vi "Generate And Open Html.vi"(8 "error in":errorcluster, 10 "Generated File Path":path, 11 "Open Generated Document":bool=TRUE) -> (0 "error out":errorcluster)   [LabVIEW 2019, in "Panther Dashboard.lvlib"]
uses:
  Panther Dashboard.lvlib
  <vilib>/Wovalab/AsciiDoc for LabVIEW/Output Format--enum.ctl
  <vilib>/Wovalab/AsciiDoc for LabVIEW/Wovalab_lib_AsciiDoctor.lvlib
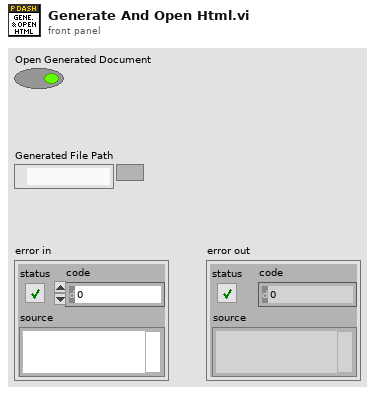
[diagram p1: front panel]
types:
  T1 = typedef "Wovalab_lib_AsciiDoctor.lvlib/Output Format--enum.ctl" = enum16{"HTML5", "PDF"}
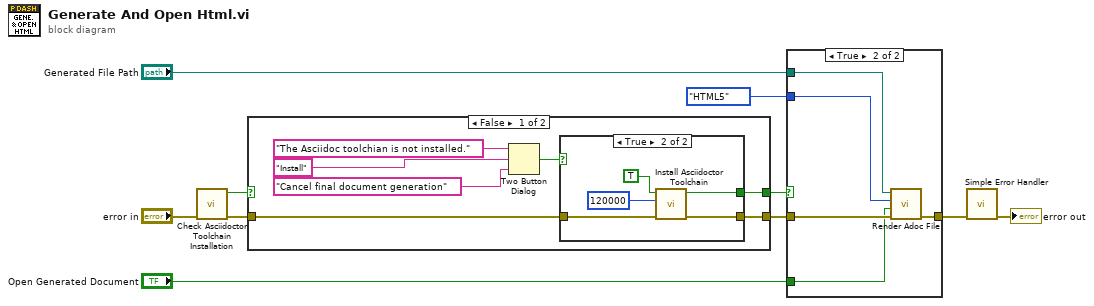
[diagram p0: block diagram]
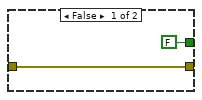
[diagram p3: hidden frame]
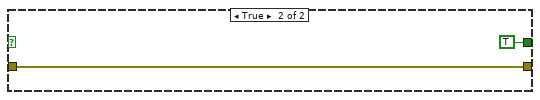
[diagram p4: hidden frame]
diagram:
  n1 = call <vilib>:"Check Asciidoctor Toolchain Installation.vi"("error in"="error in") -> ("error out"=w9:errorcluster, "Installation Ok?"=w3:bool)  [unwired: 8 in, 1 out]
  n2 = case shown="False" w3 {
    tunnel: w9 -> [w17 w26]
    tunnel: [w16 w26] -> w8
    tunnel: [w11 TRUE ("Successfull?")] -> w2
    frame False {
      n3 = Two Button Dialog(message="The Asciidoc toolchian is not installed.", 1:"Cancel final document generation" ("F button name (\"Cancel\")"), 2:"Install" ("T button name (\"OK\")")) -> (T button?=w12:bool)
      n4 = case shown="True" w12 {
        tunnel: w17 -> [w19 w24]
        tunnel: [w19 w23] -> w16
        tunnel: [FALSE ("Successfull?") w20] -> w11
        frame False {
        }
        frame True {
          n5 = call <vilib>:"Install Asciidoctor Toolchain.vi"("error in"=w24, "Dowload Timeout (60000ms)"=u32 120000, "Verbose"=TRUE) -> ("error out"=w23:errorcluster, "Successfull?"=w20:bool)  [unwired: 6 in, 1 out]
        }
      }
    }
    frame True {
    }
  }
  n6 = case shown="True" w2 {
    tunnel: [w27 w32] -> w6
    tunnel: "Generated File Path" -> [_ w30]
    tunnel: Output_Format--enum."HTML5" ("Output Format") -> [_ w29]
    tunnel: w8 -> [w27 w31]
    tunnel: "Open Generated Document" -> [_ w28]
    frame False {
    }
    frame True {
      n7 = call <vilib>:"Render Adoc File.vi"("error in"=w31, "Open Generated Document"=w28, "Output Format"=w29, "Adoc File Path"=w30) -> ("error out"=w32:errorcluster)  [unwired: 5 in, 2 out]
    }
  }
  n8 = call <vilib>:"Simple Error Handler.vi"("error in (no error)"=w6) -> ("error out"=→"error out":errorcluster)  [unwired: 4 in, 4 out]
